vi "GetControlValues.vi"(6 "error in":errorcluster, 9 "VI Refnum":refnum<vi>) -> (0 "error out":errorcluster, 4 "outputs":string[](array[string]), 5 "inputs":string[](array[string]))   [LabVIEW 2014]
uses:
  <vilib>/Utility/traverseref.llb/TRef TravTarget.ctl
  <vilib>/Utility/traverseref.llb/VI Scripting - Traverse.lvlib
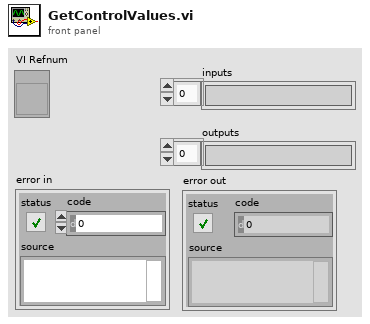
[diagram p1: front panel]
types:
  T1 = typedef "TRef TravTarget.ctl" = enum16{"FP", "BD", "Other"}
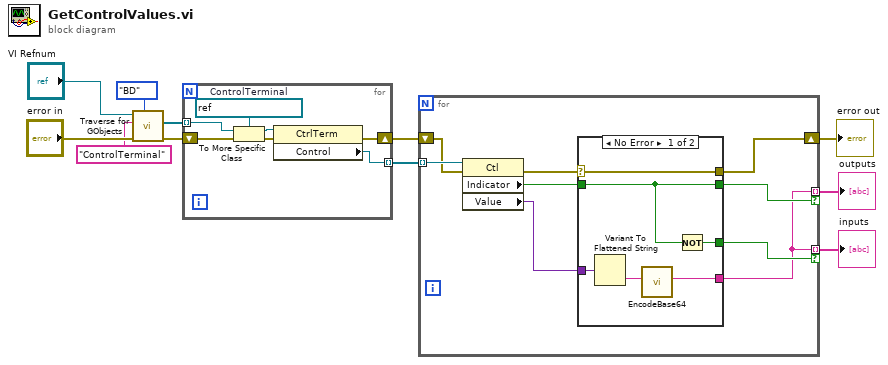
[diagram p0: block diagram]
diagram:
  n1 = call <vilib>:"Traverse for GObjects.vi"("Traverse Target"=TRef_TravTarget."BD", "error in (no error)"="error in", "Class Name"="ControlTerminal", "VI Refnum"="VI Refnum") -> ("error out"=w4:errorcluster, "References"=w5:refnum<vi>[])  [unwired: 4 in, 2 out]
  n2 = for {
    tunnel: w5 -> [w18] mode=indexing
    tunnel: [w14] -> w11 mode=indexing
    shift-right: [w13] -> w3
    shift-left: w4 -> [w12]
    w17 = refnum<vi> refnum  # ControlTerminal
    n3 = To More Specific Class(target class=w17, reference=w18, error in=w12) -> (specific class reference=w16:refnum<vi>, error out=w15:errorcluster)
    n4 = property class="CtrlTerm"(reference=w16, error in=w15) -> (error out=w13:errorcluster, "Control"=w14:refnum<vi>)  [unwired: 1 out]
  }
  n5 = for {
    tunnel: w11 -> [w27] mode=indexing
    tunnel: [w20] -> w9 mode=indexing if=w22
    tunnel: [w20] -> w8 mode=indexing if=w21
    shift-right: [w19] -> w1
    shift-left: w3 -> [w26]
    n6 = property class="Ctl"(reference=w27, error in=w26) -> (error out=w24:errorcluster, "Indicator"=w23:bool, "Value"=w25:variant)  [unwired: 1 out]
    n7 = case shown="No Error" w24 {
      selector: w24 -> [w28 w34]
      tunnel: w25 -> [w32 _]
      tunnel: w23 -> [w31 _]
      tunnel: [w31 _] -> w22
      tunnel: [w30 _] -> w21
      tunnel: [w29 _] -> w20
      tunnel: [w28 w34] -> w19
      frame No Error {
        n8 = Variant To Flattened String(Variant=w32) -> (data string=w33:string)  [unwired: 1 out]
        n9 = call "EncodeBase64.vi"("string"=w33) -> ("base64 string"=w29:string)  [unwired: 10 in]
        n10 = Not(x=w31) -> (.not. x?=w30:bool)
      }
      frame Error {
      }
    }
  }
  "error out" <- w1
  "outputs" <- w9
  "inputs" <- w8
